vi "GPIB Address Translate.vi"(1 "GPIB Address":u32=6 max=31 step=1) -> (0 "GPIB Address String":string)   [LabVIEW 2020]
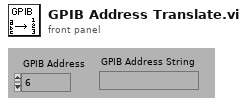
[diagram p1: front panel]
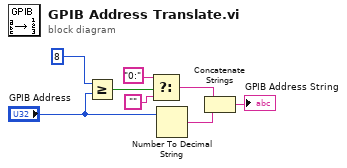
[diagram p0: block diagram]
diagram:
  n1 = Greater Or Equal?(x=u32 8, y="GPIB Address") -> (x >= y?=w8:bool)
  n2 = Select(t="0:", s=w8, f="") -> (s? t:f=w2:string)
  n3 = Number To Decimal String(number="GPIB Address") -> (decimal integer string=w3:string)  [unwired: 1 in]
  n4 = Concatenate Strings(w2, w3) -> (→"GPIB Address String":string)
